vi "SVPWMabcFXP.vi"(0 "A":fxp<+/-,32,4>, 1 "SVPWMparams":T1={"max"=0.999969482421875, "Period"=0, "Deadtime"=1}, 5 "B":fxp<+/-,32,4>, 7 "C":fxp<+/-,32,4>, 9 "input valid":bool=TRUE, 12 "enable":bool=TRUE) -> (4 "SwitchPositions":T2, 14 "Sector":u8, 15 "ready for input":bool)   [LabVIEW 2015, in "SVPWM.lvlib"]
uses:
  SVPWM.lvlib
  SwitchPositions.ctl
  SVPWM_FXP.ctl
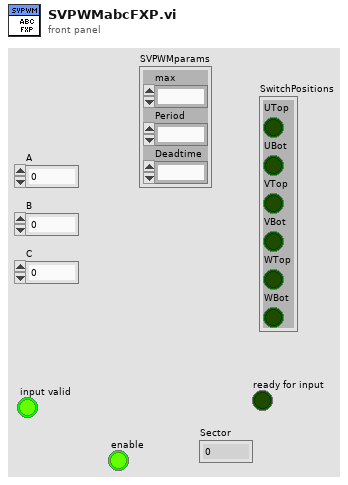
[diagram p1: front panel]
types:
  T1 = typedef "SVPWM.lvlib/SVPWM_FXP.ctl" = cluster{"max":fxp<+/-,32,4>, "Period":u32, "Deadtime":u8}
  T2 = typedef "SVPWM.lvlib/SwitchPositions.ctl" = cluster{"UTop":bool, "UBot":bool, "VTop":bool, "VBot":bool, "WTop":bool, "WBot":bool}
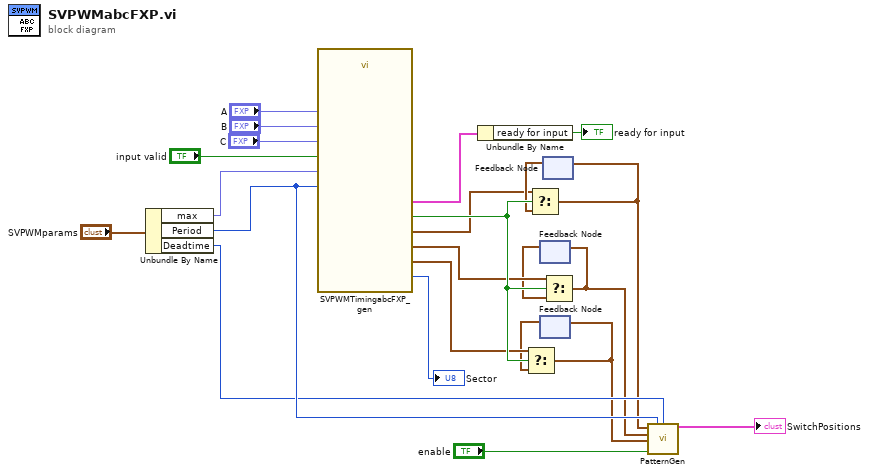
[diagram p0: block diagram]
diagram:
  n1 = Unbundle By Name("SVPWMparams") -> ("max"=w8:fxp<+/-,32,4>, "Period"=w7:u32, "Deadtime"=w6:u8)
  n2 = call "SVPWMTimingabcFXP_gen.vi"("C"="C", "A"="A", "B"="B", "Period"=w7, "input valid"="input valid", "max"=w8) -> ("Sector"=→"Sector":u8, "W_timing"=w21:cluster{"ON":u32, "OFF":u32}, "V_Timing"=w22:cluster{"ON":u32, "OFF":u32}, "output valid"=w23:bool, "feedback signals"=w11:cluster{"ready for input":bool}, "U_Timing"=w5:cluster{"ON":u32, "OFF":u32})  [unwired: 4 in]
  n3 = Unbundle By Name(w11) -> ("ready for input"=→"ready for input":bool)
  n4 = feedback #1() -> (w20:cluster{"ON":u32, "OFF":u32})  [unwired: 1 in]
  n5 = feedback #2() -> (w19:cluster{"ON":u32, "OFF":u32})  [unwired: 1 in]
  n6 = Select(t=w21, s=w23, f=w19) -> (s? t:f=w1:cluster{"ON":u32, "OFF":u32})
  n7 = feedback-in #2(w1) -> ()
  n8 = feedback #3() -> (w18:cluster{"ON":u32, "OFF":u32})  [unwired: 1 in]
  n9 = Select(t=w5, s=w23, f=w18) -> (s? t:f=w3:cluster{"ON":u32, "OFF":u32})
  n10 = feedback-in #3(w3) -> ()
  n11 = Select(t=w22, s=w23, f=w20) -> (s? t:f=w2:cluster{"ON":u32, "OFF":u32})
  n12 = feedback-in #1(w2) -> ()
  n13 = call "PatternGen.vi"("U_timing"=w3, "Period"=w7, "Deadtime"=w6, "V_timing"=w2, "W_timing"=w1, "enable"="enable") -> ("SwitchPositions"=→"SwitchPositions":T2)  [unwired: 9 in]
